vi "Send to Parent.vi"(7 "High Priority (F)":bool, 8 "error in (no error)":errorcluster, 9 "Data":variant, 10 "Message ID":string, 11 "Module in":refnum<class "Module.lvclass">) -> (0 "error out":errorcluster, 3 "Module out":refnum<class "Module.lvclass">)   [LabVIEW 2020, in "Volatus.lvlib" / "Module.lvclass"]
uses:
  Module.lvclass
  Module.lvclass/Module.ctl
  MessageQ/MessageQ.lvclass/MessageQ.ctl
  MessageQ/MessageQ.lvclass
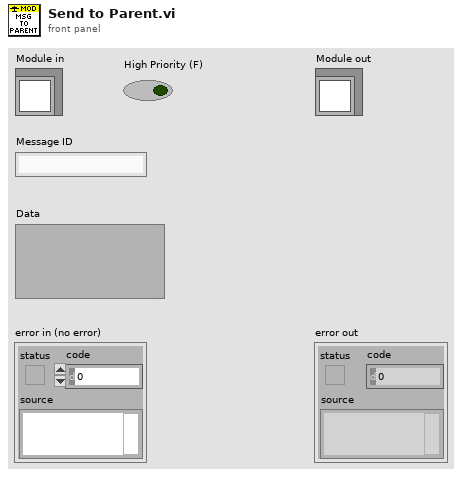
[diagram p1: front panel]
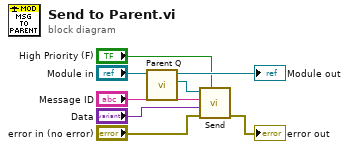
[diagram p0: block diagram]
diagram:
  n1 = call "Parent Q.vi"("Module in"="Module in") -> ("Parent Q"=w6:refnum<class "MessageQ.lvclass">, "Module out"=→"Module out":refnum<class "Module.lvclass">)  [unwired: 9 in]
  n2 = call "Send.vi"("High Priority (F)"="High Priority (F)", "error in (no error)"="error in (no error)", "Data"="Data", "ID"="Message ID", "MessageQ in"=w6) -> ("error out"=→"error out":errorcluster)  [unwired: 5 in, 1 out]
